vi "Data_Acc_Timestamp.vi"() -> ()   [LabVIEW 2009]
uses:
  <vilib>/DAQmx/read.llb/DAQmx Read.vi
  <vilib>/DAQmx/read.llb/DAQmx Read (Analog 1D Wfm NChan NSamp).vi
panel:
  in  "command line":string="ConsoleDemo.exe"
  in  "Path":path
  out "Waveform Graph":waveform(dbl)[](graph)
  in  "?":bool
  in  "File Name":path=path "C:/Users/Preetham/Documents/PhD Workspace/LabVIEW Stuffs/Data Write/LVDT Write/Output_Data.lvm"
  # "External Path for an Executable File"
  # "External Path for an Executable File"
  # "Path for a Text File"
  # "Choose a location for the LabVIEW Measurements File and then \nrun this VI."
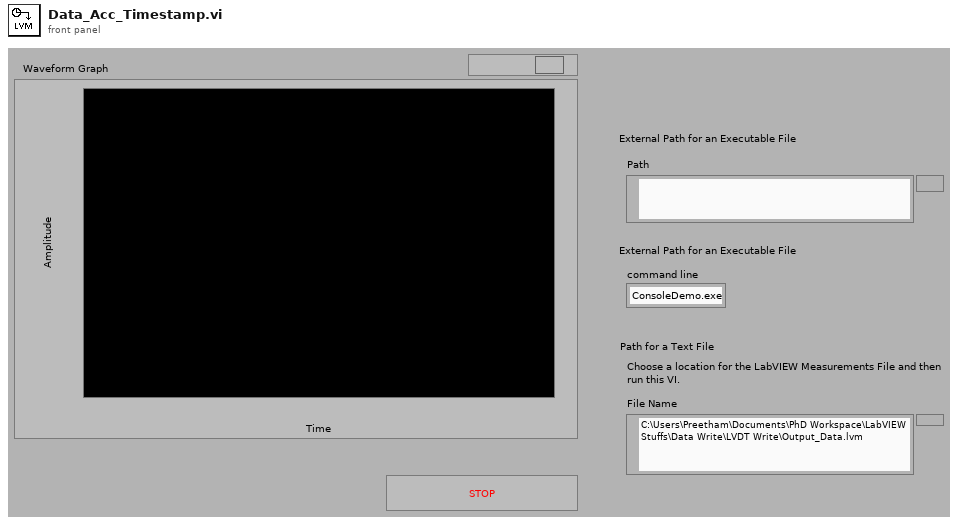
[diagram p1: front panel]
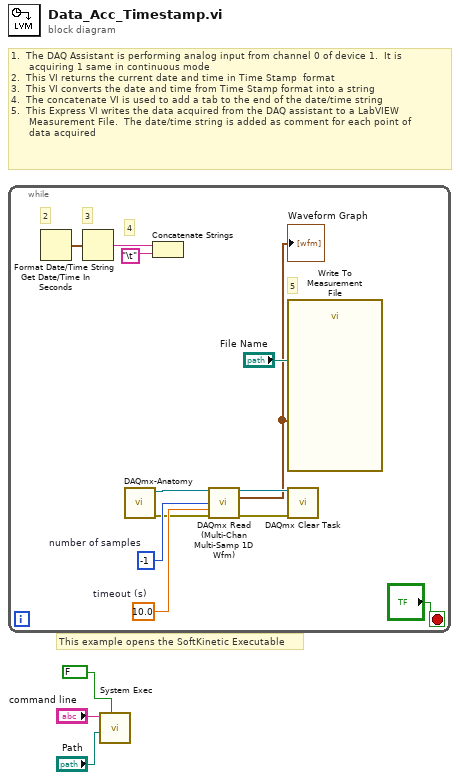
[diagram p0: block diagram]
diagram:
  # "This example opens the SoftKinetic Executable"
  # "1.  The DAQ Assistant is performing analog input from channel 0 of device 1.  It is \n      acquiring 1 same in continuous mode\n2.  This VI returns the current date and time in Time Stamp  format\n3.  This VI converts the date and time from Time Stamp format into a string\n4.  The concatenate VI is used to add a tab to the end of the date/time string\n5.  This Express VI writes the data acquired from the DAQ assistant to a LabVIEW \n      Measurement File.  The date/time string is added as comment for each point of \n      data acquired"
  n1 = while {
    stop <- "?" stop-if-true
    w9 = 10.0  # timeout (s)
    w10 = -1  # number of samples
    # "5"
    # "4"
    # "3"
    # "2"
    n2 = Get Date/Time In Seconds() -> (seconds since 1Jan1904=w13:timestamp)
    n3 = Format Date/Time String(seconds (now)=w13) -> (date/time string=w15:string)  [unwired: 2 in]
    n4 = call "DAQmx-Anatomy.vi"() -> ("error out"=w5:errorcluster, "task out"=w6:refnum<k21>)  [unwired: 10 in]
    n5 = Concatenate Strings(w15, "\t") -> ()  [unwired: 1 out]
    n6 = call-poly "DAQmx Read (Multi-Chan Multi-Samp 1D Wfm).vi"("task/channels in"=w6, "number of samples per channel"=w10, "timeout"=w9, "error in"=w5) -> ("task out"=w7:refnum<k21>, "data"=w4:waveform(dbl)[], "error out"=w8:errorcluster)  [unwired: 9 out]
    "Waveform Graph" <- w4
    n7 = call "Write To Measurement File"("Signals"=w4, "Filename"="File Name") -> ()  [unwired: 15 in, 3 out]
    n8 = call <vilib>:"DAQmx Clear Task.vi"("task in"=w7, "error in"=w8) -> ()  [unwired: 14 out]
  }
  n9 = call <vilib>:"System Exec.vi"("wait until completion? (T)"=FALSE, "working directory"="Path", "command line"="command line") -> ()  [unwired: 5 in, 4 out]
